vi "ReCheck Increment Limits.vi"(8 "error in (no error)":errorcluster, 11 "LBCB Number":T1) -> (0 "error out":errorcluster)   [LabVIEW 2009]
uses:
  Data Access Objects/Metadata/LBCB Number.ctl
  Data Access Objects/Metadata/Persistant DAO Actions.ctl
  Limits/Within Limits Matrix.ctl
  Limits/Actuator Faults.ctl
  Limits/Cart Disp Faults.ctl
  Limits/Cart Force Faults.ctl
  Control Loop/Act & Cart Commands.ctl
  Data Access Objects/Metadata/DAO Actions.ctl
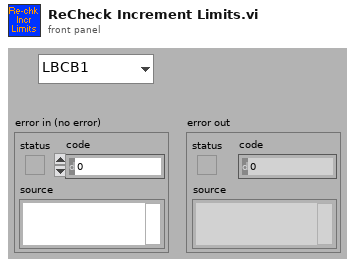
[diagram p1: front panel]
types:
  T1 = typedef "LBCB Number.ctl" = enum16{"LBCB1", "LBCB2"}
  T2 = typedef "DAO Actions.ctl" = enum16{"Init", "Get", "Set"}
  T3 = typedef "Act & Cart Commands.ctl" = cluster{"Act Cmd":dbl[], "Cart Cmd":dbl[]}
  T4 = typedef "Within Limits Matrix.ctl" = cluster{"Act Disp":T5, "Act Force":T5, "Act Incr":T5, "Cart Disp":T6, "Cart Force":T7, "Cart Incr":T6}
  T5 = typedef "Actuator Faults.ctl" = cluster{"X1":bool, "X2":bool, "Y1":bool, "Z1":bool, "Z2":bool, "Z3":bool}
  T6 = typedef "Cart Disp Faults.ctl" = cluster{"Dx":bool, "Dy":bool, "Dz":bool, "Rx":bool, "Ry":bool, "Rz":bool}
  T7 = typedef "Cart Force Faults.ctl" = cluster{"Fx":bool, "Fy":bool, "Fz":bool, "Mx":bool, "My":bool, "Mz":bool}
  T8 = typedef "Persistant DAO Actions.ctl" = enum16{"Init", "Get", "Set", "Load", "Save"}
  T9 = typedef "Actuator Point.ctl" = cluster{"X1":dbl, "X2":dbl, "Y1":dbl, "Z1":dbl, "Z2":dbl, "Z3":dbl}
  T10 = typedef "Cartesian Point.ctl" = cluster{"Dx":dbl, "Dy":dbl, "Dz":dbl, "Rx":dbl, "Ry":dbl, "Rz":dbl}
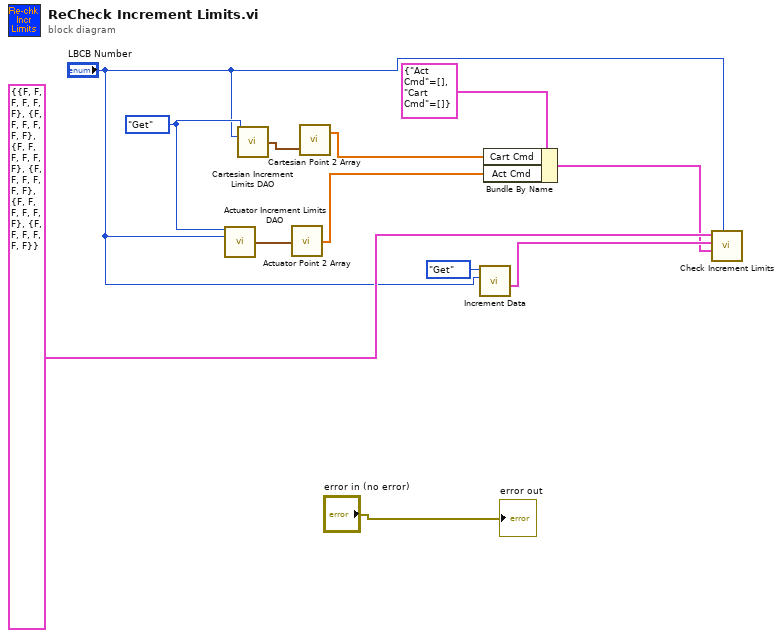
[diagram p0: block diagram]
diagram:
  w12 = Persistant_DAO_Actions."Get" ("Actions")
  n1 = call "Actuator Increment Limits DAO.vi"("Actions"=w12, "LBCB Number"="LBCB Number") -> ("Inc Limits Out"=w9:T9)  [unwired: 11 in, 2 out]
  n2 = call "Cartesian Increment Limits DAO.vi"("Actions"=w12, "LBCB Number"="LBCB Number") -> ("Inc Limits Out"=w10:T10)  [unwired: 11 in, 2 out]
  n3 = call "Actuator Point 2 Array.vi"("Actuator Point"=w9) -> ("Array"=w6:dbl[])
  n4 = call "Cartesian Point 2 Array.vi"("Cart Disp"=w10) -> ("Array"=w7:dbl[])  [unwired: 2 in]
  n5 = call "Increment Data.vi"("LBCB Number"="LBCB Number", "DAO Actions"=DAO_Actions."Get") -> ("Increments Out"=w2:T3)  [unwired: 8 in, 1 out]
  n6 = Bundle By Name(cluster=T3 {"Act Cmd"=[], "Cart Cmd"=[]} ("Increments Out"), "Cart Cmd"=w7, "Act Cmd"=w6) -> (w1:T3)
  n7 = call "Check Increment Limits.vi"("LBCB Number"="LBCB Number", "Increment Limits"=w1, "Increments In"=w2, "Within Limits In"=T4 {"Act Disp"={"X1"=FALSE, "X2"=FALSE, "Y1"=FALSE, "Z1"=FALSE, "Z2"=FALSE, "Z3"=FALSE}, "Act Force"={"X1"=FALSE, "X2"=FALSE, "Y1"=FALSE, "Z1"=FALSE, "Z2"=FALSE, "Z3"=FALSE}, "Act Incr"={"X1"=FALSE, "X2"=FALSE, "Y1"=FALSE, "Z1"=FALSE, "Z2"=FALSE, "Z3"=FALSE}, "Cart Disp"={"Dx"=FALSE, "Dy"=FALSE, "Dz"=FALSE, "Rx"=FALSE, "Ry"=FALSE, "Rz"=FALSE}, "Cart Force"={"Fx"=FALSE, "Fy"=FALSE, "Fz"=FALSE, "Mx"=FALSE, "My"=FALSE, "Mz"=FALSE}, "Cart Incr"={"Dx"=FALSE, "Dy"=FALSE, "Dz"=FALSE, "Rx"=FALSE, "Ry"=FALSE, "Rz"=FALSE}}) -> ()  [unwired: 2 in, 4 out]
  "error out" <- "error in (no error)"
